vi "Next State.vi"(8 "error in (no error)":errorcluster, 10 "New_State":u32, 11 "State Machine in":refnum<class "State Machine.lvclass">) -> (0 "error out":errorcluster, 3 "State Machine out":refnum<class "State Machine.lvclass">)   [LabVIEW 2018, in "State Machine.lvclass"]
uses:
  State Machine.lvclass
  State Machine.lvclass/State Machine.ctl
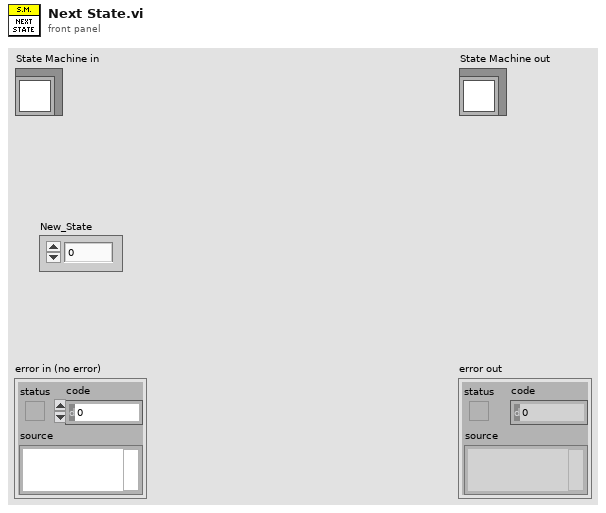
[diagram p1: front panel]
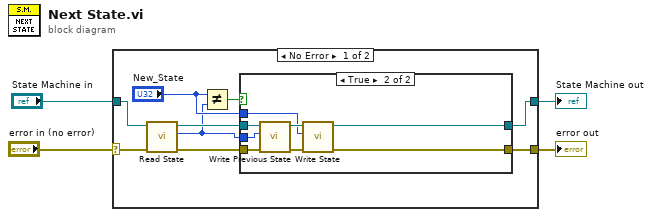
[diagram p0: block diagram]
diagram:
  n1 = case shown="No Error" "error in (no error)" {
    selector: "error in (no error)" -> [w9 w25]
    tunnel: [w11 w25] -> w1
    tunnel: [w13 w24] -> w2
    tunnel: "State Machine in" -> [w8 w24]
    frame No Error {
      n2 = call "Read State.vi"("error in (no error)"=w9, "State Machine in"=w8) -> ("error out"=w7:errorcluster, "State"=w5:u16, "State Machine out"=w6:refnum<class "State Machine.lvclass">)  [unwired: 7 in]
      n3 = Not Equal?(x="New_State", y=w5) -> (x != y?=w12:bool)
      n4 = case shown="True" w12 {
        tunnel: w6 -> [w15 w23]
        tunnel: [w15 w19] -> w13
        tunnel: w5 -> [_ w16]
        tunnel: "New_State" -> [_ w17]
        tunnel: [w14 w20] -> w11
        tunnel: w7 -> [w14 w22]
        frame False {
          # "ESTADO DESEJADO JÁ É O ESTADO ATUAL"
        }
        frame True {
          n5 = call "Write Previous State.vi"("error in (no error)"=w22, "Previous State"=w16, "State Machine in"=w23) -> ("error out"=w21:errorcluster, "State Machine out"=w18:refnum<class "State Machine.lvclass">)  [unwired: 7 in]
          n6 = call "Write State.vi"("error in (no error)"=w21, "State"=w17, "State Machine in"=w18) -> ("error out"=w20:errorcluster, "State Machine out"=w19:refnum<class "State Machine.lvclass">)  [unwired: 7 in]
        }
      }
    }
    frame Error {
    }
  }
  "error out" <- w1
  "State Machine out" <- w2
